vi "accelcalc2.vi"(1 "Y":dbl, 2 "Z":dbl, 8 "error in (no error)":errorcluster) -> (9 "Result":dbl, 10 "error out":errorcluster)   [LabVIEW 2017]
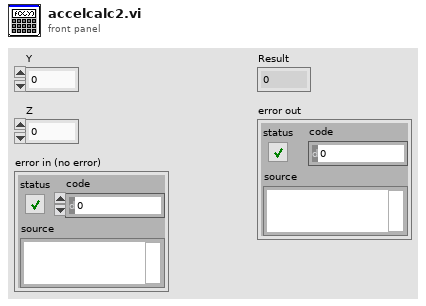
[diagram p1: front panel]
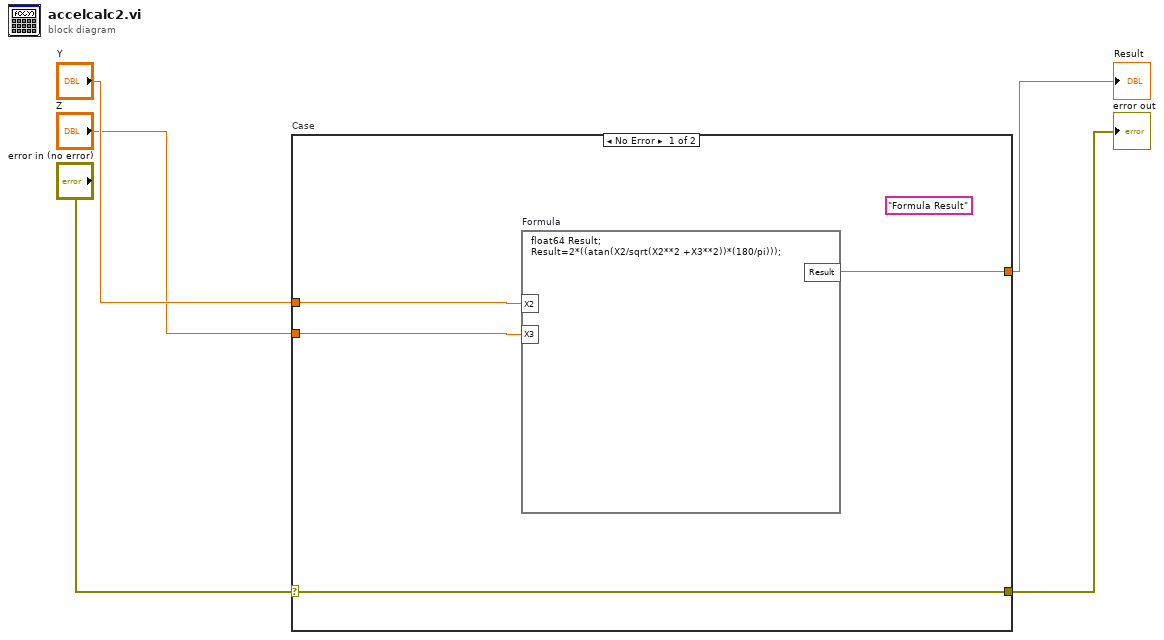
[diagram p0: block diagram]
diagram:
  n1 = case "Case" shown="No Error" "error in (no error)" {
    selector: "error in (no error)" -> [w6 w10]
    tunnel: [w7 _] -> w2
    tunnel: [w6 w10] -> w1
    tunnel: "Y" -> [w9 _]
    tunnel: "Z" -> [w8 _]
    frame No Error {
      (unwired) "Formula Result" ("Name Modifier")
      n2 = formula code="float64 Result;\nResult=2*((atan(X2/sqrt(X2**2 +X3**2))*(180/pi)));"("X2"=w9, "X3"=w8) -> ("Result"=w7:dbl)
    }
    frame Error {
    }
  }
  "Result" <- w2
  "error out" <- w1
